vi "XY Graph Check-Uncheck Menu Items.vi"(8 "Error In":errorcluster, 9 "Coords":T2, 10 "Menu in":refnum<k9>, 11 "XY Graph Refnum":T3) -> (0 "Error Out (dup)":errorcluster, 1 "Click Location":T1)   [LabVIEW 2019, in "XY Graph Add-Ons.lvlib"]
uses:
  XY Graph Add-Ons.lvlib
  XY Graph Refnum.ctl
  <vilib>/Utility/miscctls.llb/LVPoint32TypeDef.ctl
  XY Graph Click Location.ctl
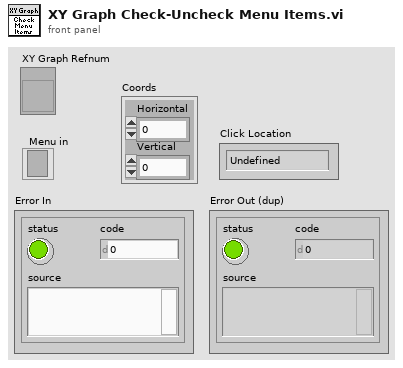
[diagram p1: front panel]
types:
  T1 = typedef "XY Graph Click Location.ctl" = enum16{"Undefined", "Plot Area", "Plot Legend", "Scale Legend", "Graph Palette", "Cursor Legend", "Graph Border"}
  T2 = typedef "LVPoint32TypeDef.ctl" = cluster{"Horizontal":i32, "Vertical":i32}
  T3 = typedef "XY Graph Add-Ons.lvlib/XY Graph Refnum.ctl" = refnum<vi>
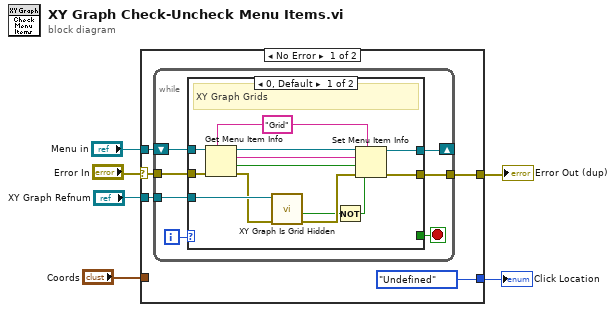
[diagram p0: block diagram]
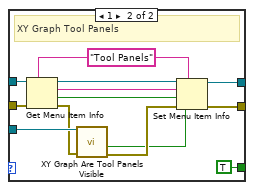
[diagram p2: hidden frame]
diagram:
  n1 = case shown="No Error" "Error In" {
    selector: "Error In" -> [w10 w45]
    tunnel: "XY Graph Refnum" -> [w9 _]
    tunnel: "Menu in" -> [w11 _]
    tunnel: "Coords" -> [_ _]
    tunnel: [XY_Graph_Click_Location."Undefined" ("Click Location") _] -> w2
    tunnel: [w7 w45] -> w1
    frame No Error {
      n2 = while {
        tunnel: w9 -> [w18]
        tunnel: w10 -> [w15]
        shift-right: [w14] -> _
        shift-left: w11 -> [w17]
        tunnel: [w12] -> w7
        i -> [w16]
        stop <- w13 stop-if-true
        n3 = case shown="0, Default" w16 {
          tunnel: w18 -> [w31 w37]
          tunnel: w17 -> [w30 w44]
          tunnel: w15 -> [w28 w43]
          tunnel: [w20 w38] -> w14
          tunnel: [_ TRUE] -> w13
          tunnel: [w19 w32] -> w12
          frame 0, Default {
            w21 = "Grid" ("item tag")
            # "XY Graph Grids"
            n4 = Get Menu Item Info(7:w21, 8:w28, 11:w30) -> (0:w29:errorcluster, 1:w23:bool, 2:w22:string, 3:w27:refnum<k9>)  [unwired: 3 out]
            n5 = call "XY Graph Is Grid Hidden.vi"("Error In"=w29, "XY Graph Ref"=w31) -> ("Error Out (dup)"=w26:errorcluster, "Hidden Grid(s)"=w25:bool)  [unwired: 7 in, 1 out]
            n6 = Not(x=w25) -> (.not. x?=w24:bool)
            n7 = Set Menu Item Info(6:w24, 7:w21, 8:w26, 9:w23, 10:w22, 11:w27) -> (0:w19:errorcluster, 3:w20:refnum<k9>)  [unwired: 1 in]
          }
          frame 1 {
            w39 = "Tool Panels" ("item tag")
            # "XY Graph Tool Panels"
            n8 = Get Menu Item Info(7:w39, 8:w43, 11:w44) -> (0:w36:errorcluster, 1:w41:bool, 2:w40:string, 3:w42:refnum<k9>)  [unwired: 3 out]
            n9 = call "XY Graph Are Tool Panels Visible.vi"("Error In"=w36, "XY Graph Ref"=w37) -> ("Error Out"=w35:errorcluster, "Any Panel Visible?"=w34:bool)  [unwired: 7 in, 1 out]
            n10 = Set Menu Item Info(6:w34, 7:w39, 8:w35, 9:w41, 10:w40, 11:w42) -> (0:w32:errorcluster, 3:w38:refnum<k9>)  [unwired: 1 in]
          }
        }
      }
    }
    frame Error {
    }
  }
  "Error Out (dup)" <- w1
  "Click Location" <- w2
